vi "Get Request Type.vi"(8 "error in (no error)":errorcluster, 11 "GetInputVolume in":refnum<class "GetInputVolume.lvclass">) -> (0 "error out":errorcluster, 2 "Request Type":string, 3 "GetInputVolume out":refnum<class "GetInputVolume.lvclass">)   [LabVIEW 2022 SP3, in "obs-websocket-lv.lvlib" / "GetInputVolume.lvclass"]
uses:
  GetInputVolume.lvclass
  GetInputVolume.lvclass/GetInputVolume.ctl
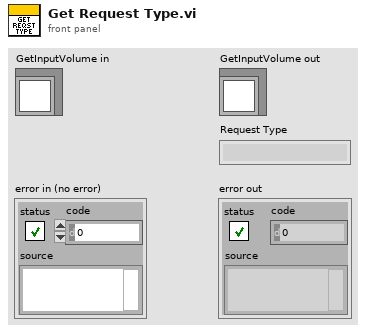
[diagram p1: front panel]
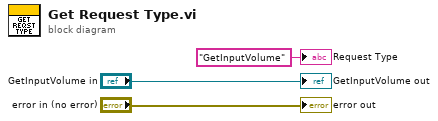
[diagram p0: block diagram]
diagram:
  "error out" <- "error in (no error)"
  "GetInputVolume out" <- "GetInputVolume in"
  "Request Type" <- "GetInputVolume" ("Request Type")
